vi "GetFixedName.vi"(6 "error in":errorcluster, 9 "SubVI in":refnum<class "SubVI.lvclass">) -> (0 "error out":errorcluster, 3 "SubVI out":refnum<class "SubVI.lvclass">, 4 "fixed name":string)   [LabVIEW 2014, in "SubVI.lvclass"]
uses:
  SubVI.lvclass
  SubVI.lvclass/SubVI.ctl
  Python/Parsing/Python Functions.lvlib
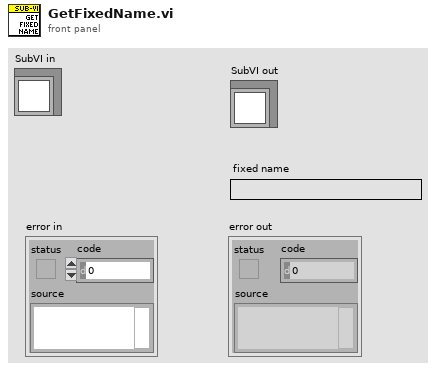
[diagram p1: front panel]
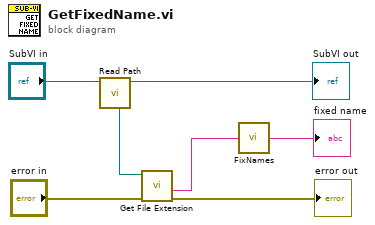
[diagram p0: block diagram]
diagram:
  n1 = call "Read Path.vi"("SubVI in"="SubVI in") -> ("SubVI out"=→"SubVI out":refnum<class "SubVI.lvclass">, "Path"=w4:path)  [unwired: 7 in]
  n2 = call <vilib>:"Get File Extension.vi"("error in (no error)"="error in", "file"=w4) -> ("error out"=→"error out":errorcluster, "filename without extension"=w3:string)  [unwired: 6 in, 2 out]
  n3 = call "FixNames.vi"("name"=w3) -> ("python name"=→"fixed name":string)
